vi "Read String Configuration.vi"(8 "error in (no error)":errorcluster, 9 "Default If Not Found":string, 10 "Name":string, 11 "IniFileSection in":refnum<class "IniFileSection.lvclass">) -> (0 "error out":errorcluster, 1 "Not Found?":bool, 2 "Value":string, 3 "IniFileSection out":refnum<class "IniFileSection.lvclass">)   [LabVIEW 2017, in "IniFileSection.lvclass"]
uses:
  IniFileSection.lvclass
  IniFileSection.lvclass/IniFileSection.ctl
  <vilib>/Utility/config.llb/Read Key (String).vi
  <vilib>/Utility/config.llb/NI_LVConfig.lvlib
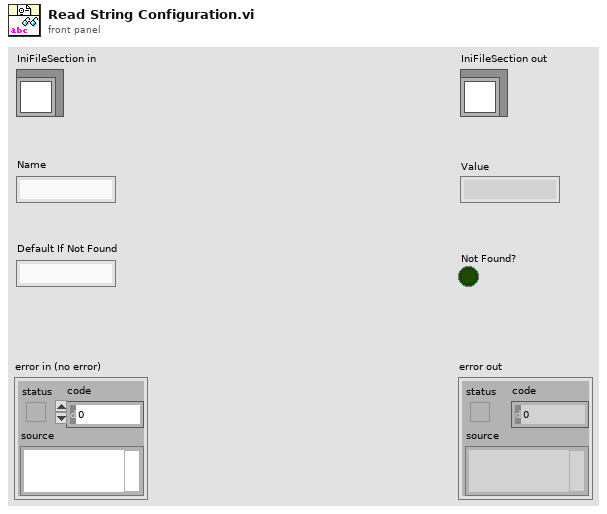
[diagram p1: front panel]
types:
  T1 = typedef "NI_LVConfig.lvlib/Config Data RefNum.ctl" = refnum<k1>
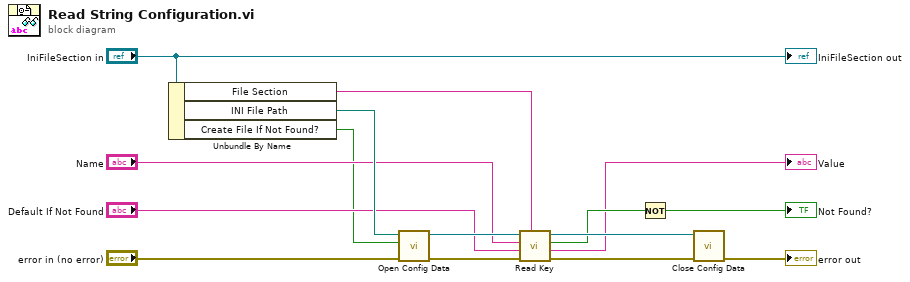
[diagram p0: block diagram]
diagram:
  n1 = Unbundle By Name("IniFileSection in") -> ("File Section"=w9:string, "INI File Path"=w10:path, "Create File If Not Found?"=w1:bool)
  n2 = call <vilib>:"Open Config Data.vi"("error in (no error)"="error in (no error)", "create file if necessary (T)"=w1, "configuration file path"=w10) -> ("error out"=w15:errorcluster, "refnum"=w13:T1)  [unwired: 6 in, 1 out]
  n3 = call-poly <vilib>:"Read Key.vi"("section"=w9, "error in (no error)"=w15, "default value"="Default If Not Found", "key"="Name", "refnum"=w13) -> ("error out"=w14:errorcluster, "value"=→"Value":string, "found?"=w11:bool, "refnum out"=w12:T1)  [unwired: 3 in]
  n4 = Not(x=w11) -> (.not. x?=→"Not Found?":bool)
  n5 = call <vilib>:"Close Config Data.vi"("error in (no error)"=w14, "refnum"=w12) -> ("error out"=→"error out":errorcluster)  [unwired: 8 in, 1 out]
  "IniFileSection out" <- "IniFileSection in"
